vi "Verify.vi"(8 "error in":errorcluster, 10 "Test Data":string, 11 "TestCase":refnum<class "TestCase.lvclass">) -> (0 "error out":errorcluster, 3 "TestCase":refnum<class "TestCase.lvclass">)   [LabVIEW 2020, in "VITester.Extension.lvlib"]
uses:
  VITester.Extension.lvlib
  Approval Tests/Approval Tests.lvlib
  <vilib>/addons/_JKI Toolkits/VI Tester/TestCase.llb/TestCase.lvclass
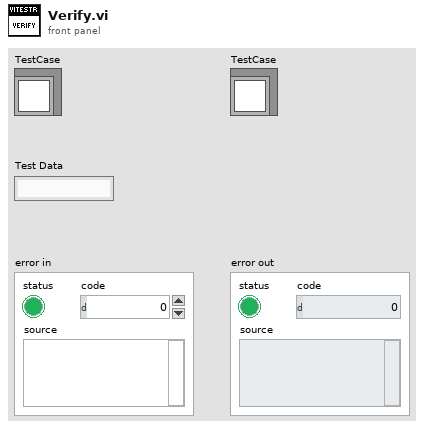
[diagram p1: front panel]
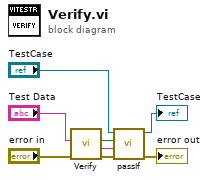
[diagram p0: block diagram]
diagram:
  n1 = call "Verify.vi"("error in"="error in", "Test Data"="Test Data") -> ("error out"=w6:errorcluster, "Failure Message"=w1:string, "Passed?"=w2:bool)  [unwired: 7 in]
  n2 = call-dynamic "passIf.vi"("error in (no error)"=w6, "message (\"\")"=w1, "pass"=w2, "TestCase in"="TestCase") -> ("error out"=→"error out":errorcluster, "TestCase out"=→"TestCase":refnum<class "TestCase.lvclass">)  [unwired: 6 in]
